vi "Logger.Stats.Fglb.vi"(4 "Time To":dbl, 6 "Time From":dbl, 7 "Action (get)":T2=enum."get", 8 "error in (no error)":errorcluster, 9 "dbg_NOK":dbl[](array[numeric]), 10 "dbg_OK":dbl[](array[numeric]), 11 "Variant":string) -> (0 "error out":errorcluster, 2 "Results":T1[](array[typedef]) {"Time From" format="%<%X %x>T"; "Time To" format="%<%X %x>T"})   [LabVIEW 2016]
uses:
  Logger.Stats.Fglb.Action.ctl
  Logger.Stats.Fglb.Result.ctl
  Global/ApplicationGlobal.vi
panel:
  out "dbg_var":string[](array[string])
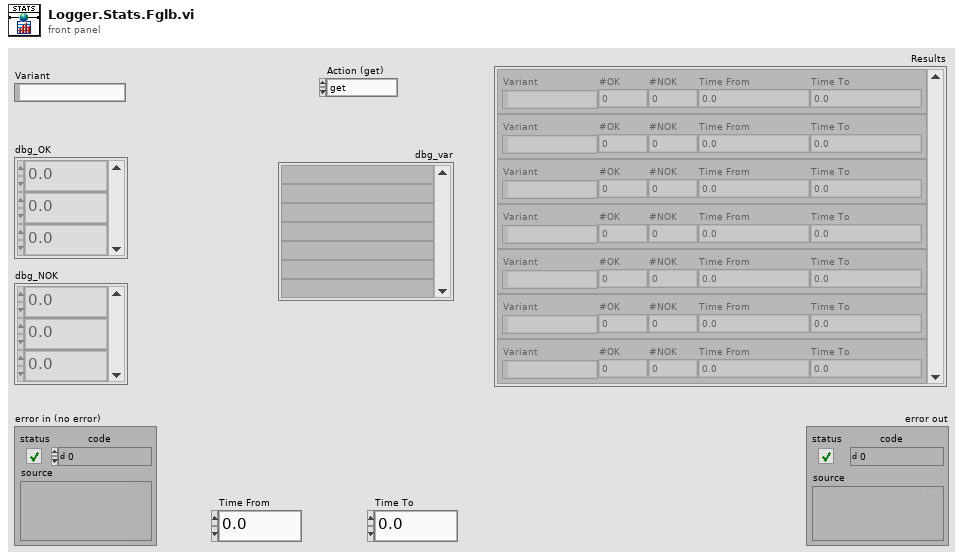
[diagram p1: front panel]
types:
  T1 = typedef "Logger.Stats.Fglb.Result.ctl" = cluster{"Variant":string, "#OK":i32, "#NOK":i32, "Time From":dbl, "Time To":dbl}
  T2 = typedef "Logger.Stats.Fglb.Action.ctl" = enum16{"init", "add", "get", "get all"}
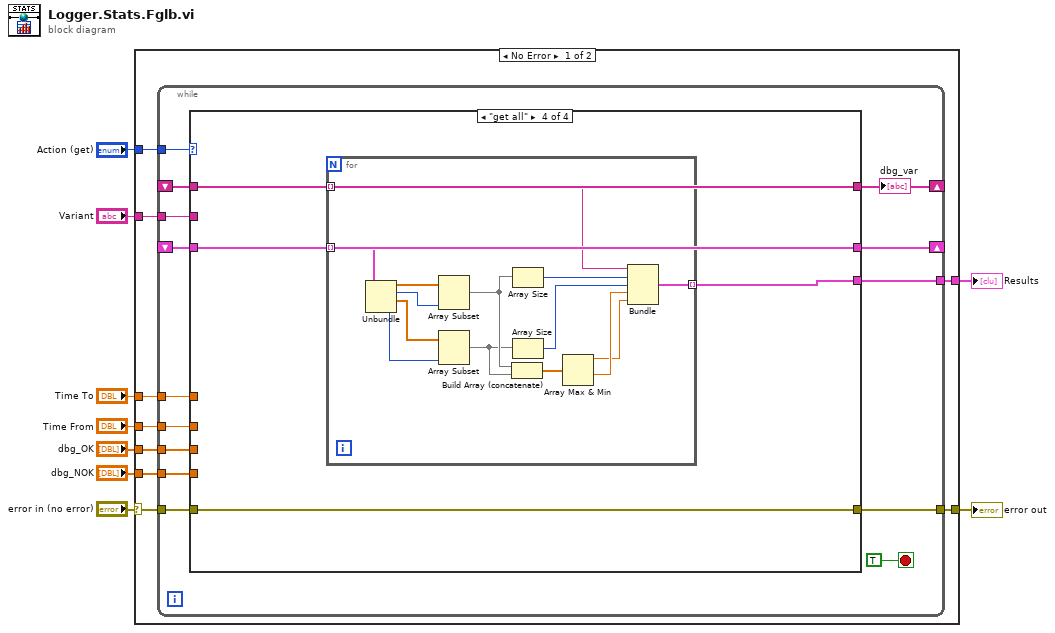
[diagram p0: block diagram]
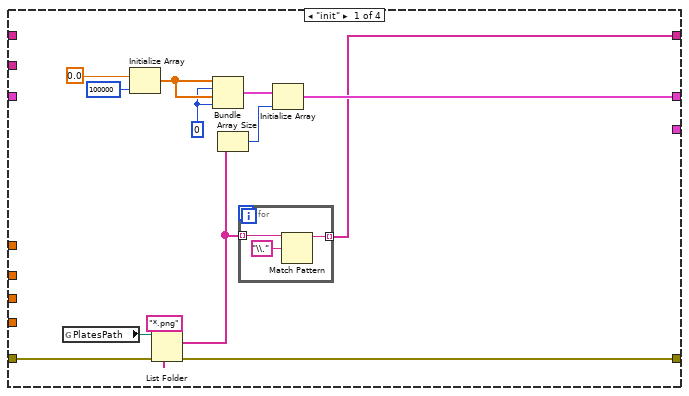
[diagram p2: hidden frame]
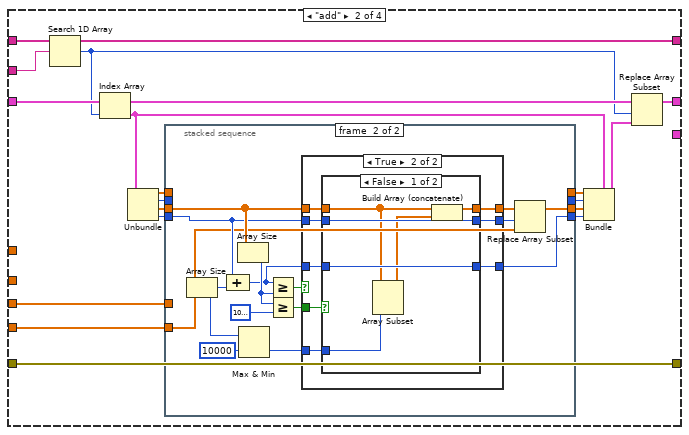
[diagram p3: hidden frame]
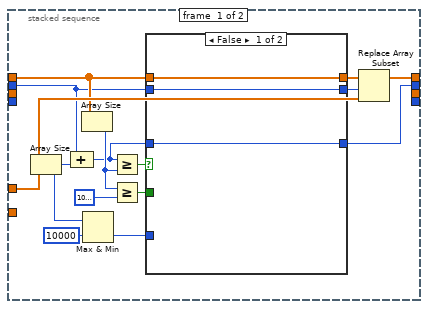
[diagram p4: hidden frame]
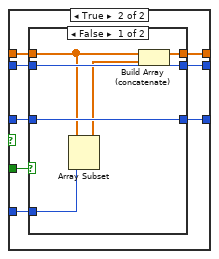
[diagram p5: hidden frame]
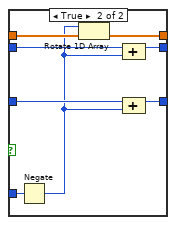
[diagram p6: hidden frame]
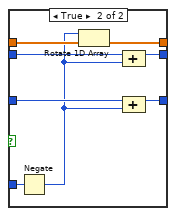
[diagram p8: hidden frame]
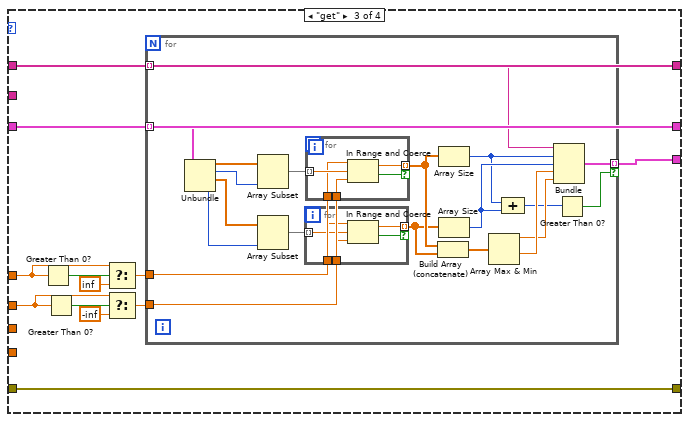
[diagram p9: hidden frame]
diagram:
  n1 = case shown="No Error" "error in (no error)" {
    selector: "error in (no error)" -> [w17 w207]
    tunnel: "Action (get)" -> [w18 _]
    tunnel: [w16 w207] -> w7
    tunnel: "Variant" -> [w15 _]
    tunnel: "dbg_OK" -> [w14 _]
    tunnel: "dbg_NOK" -> [w13 _]
    tunnel: "Time From" -> [w12 _]
    tunnel: "Time To" -> [w11 _]
    tunnel: [w10 _] -> w1
    frame No Error {
      n2 = while {
        tunnel: w18 -> [w32]
        shift-right: [w29] -> _
        shift-left: _ -> [w30]
        tunnel: w17 -> [w28]
        shift-right: [w27] -> _
        shift-left: _ -> [w26]
        tunnel: [w25] -> w16
        tunnel: w15 -> [w24]
        tunnel: w14 -> [w23]
        tunnel: w13 -> [w22]
        tunnel: w12 -> [w21]
        tunnel: w11 -> [w20]
        tunnel: [w19] -> w10
        stop <- TRUE stop-if-true
        n3 = case shown="\"get all\"" w32 {
          tunnel: w30 -> [_ w65 w147 w189]
          tunnel: [w33 w65 w147 w189] -> w29
          tunnel: w28 -> [w42 w51 w158 w192]
          tunnel: [w37 w63 w149 w191] -> w27
          tunnel: w26 -> [_ w64 w149 w191]
          tunnel: [w36 w51 w158 w192] -> w25
          tunnel: w24 -> [_ w66 _ _]
          tunnel: w23 -> [_ w58 _ _]
          tunnel: w22 -> [_ w52 _ _]
          tunnel: w21 -> [_ _ w157 _]
          tunnel: w20 -> [_ _ w152 _]
          tunnel: [_ _ w148 w190] -> w19
          frame "init" {
            w43 = 0
            n4 = global read "ApplicationGlobal.vi" "PlatesPath"() -> (w40:path)
            n5 = Initialize Array(0.0 ("Time Stamp"), 100000 ("dimension size")) -> (w44:dbl[])
            n6 = List Folder(path=w40, pattern="*.png" ("string"), error in=w42) -> (filenames=w34:string[], error out=w36:errorcluster)  [unwired: 1 in, 2 out]
            n7 = Bundle(w44, w43, w44, w43) -> (w39:cluster{dbl[], i32, dbl[], i32})  [unwired: 1 in]
            n8 = Array Size(array=w34) -> (size(s)=w38:i32)
            n9 = for {
              tunnel: w34 -> [w48] mode=indexing
              tunnel: [w46] -> w33 mode=indexing
              n10 = Match Pattern(string=w48, regular expression="\\.") -> (before substring=w46:string)  [unwired: 1 in, 3 out]
            }
            n11 = Initialize Array(w39, w38) -> (w37:cluster{dbl[], i32, dbl[], i32}[])
          }
          frame "add" {
            n12 = Search 1D Array(1D array=w65, element=w66) -> (index of element=w62:i32)  [unwired: 1 in]
            n13 = Index Array(array=w64, index=w62) -> (element=w61:cluster{dbl[], i32, dbl[], i32})
            n14 = Unbundle(w61) -> (w57:dbl[], w56:i32, w54:dbl[], w53:i32)
            n15 = stacked-sequence {
              tunnel: [w81 _] -> w59
              tunnel: w58 -> [w72 _]
              tunnel: w57 -> [w71 _]
              tunnel: w56 -> [w70 _]
              tunnel: [w73 _] -> w55
              tunnel: w54 -> [_ w109]
              tunnel: w53 -> [_ w108]
              tunnel: w52 -> [_ w107]
              tunnel: [_ w111] -> w50
              tunnel: [_ w110] -> w49
              frame #0 {
                n16 = Array Size(array=w72) -> (size(s)=w69:i32)
                n17 = Compound Arithmetic op=ADD(w70, w69) -> (w74:i32)
                n18 = Array Size(array=w71) -> (size(s)=w80:i32)
                n19 = Max & Min(x=w69, y=10000 ("dimension size")) -> (min(x,y)=w67:i32)  [unwired: 1 out]
                n20 = Greater Or Equal?(x=w74, y=w80) -> (x >= y?=w78:bool)
                n21 = Greater Or Equal?(x=w80, y=1000000) -> (x >= y?=w76:bool)
                n22 = case shown="False" w78 {
                  tunnel: w71 -> [w84 w92]
                  tunnel: [w84 w91] -> w77
                  tunnel: w76 -> [_ w90]
                  tunnel: w70 -> [w83 w89]
                  tunnel: [w83 w86] -> w75
                  tunnel: w74 -> [w82 w88]
                  tunnel: [w82 w87] -> w73
                  tunnel: w67 -> [_ w85]
                  frame False {
                  }
                  frame True {
                    n23 = case shown="False" w90 {
                      tunnel: w92 -> [w94 w106]
                      tunnel: [w98 w105] -> w91
                      tunnel: w89 -> [w96 w101]
                      tunnel: w88 -> [w97 w103]
                      tunnel: [w97 w102] -> w87
                      tunnel: [w96 w99] -> w86
                      tunnel: w85 -> [w95 w104]
                      frame False {
                        n24 = Array Subset(array=w94, length=w95) -> (w93:dbl[])  [unwired: 1 in]
                        n25 = Build Array (concatenate)(w94, w93) -> (w98:dbl[])
                      }
                      frame True {
                        n26 = Negate(x=w104) -> (-x=w100:i32)
                        n27 = Rotate 1D Array(1:w106, 2:w100) -> (0:w105:dbl[])
                        n28 = Compound Arithmetic op=ADD(w101, w100) -> (w99:i32)
                        n29 = Compound Arithmetic op=ADD(w103, w100) -> (w102:i32)
                      }
                    }
                  }
                }
                n30 = Replace Array Subset(array=w77, new element=w72, index=w75) -> (w81:dbl[])
              }
              frame #1 {
                n31 = Array Size(array=w107) -> (size(s)=w114:i32)
                n32 = Compound Arithmetic op=ADD(w108, w114) -> (w115:i32)
                n33 = Array Size(array=w109) -> (size(s)=w121:i32)
                n34 = Max & Min(x=w114, y=10000 ("dimension size")) -> (min(x,y)=w112:i32)  [unwired: 1 out]
                n35 = Greater Or Equal?(x=w115, y=w121) -> (x >= y?=w119:bool)
                n36 = Greater Or Equal?(x=w121, y=1000000) -> (x >= y?=w117:bool)
                n37 = case shown="True" w119 {
                  tunnel: w109 -> [w124 w132]
                  tunnel: [w124 w131] -> w118
                  tunnel: w117 -> [_ w130]
                  tunnel: w108 -> [w123 w129]
                  tunnel: [w123 w126] -> w116
                  tunnel: w115 -> [w122 w128]
                  tunnel: [w122 w127] -> w111
                  tunnel: w112 -> [_ w125]
                  frame False {
                  }
                  frame True {
                    n38 = case shown="False" w130 {
                      tunnel: w132 -> [w134 w146]
                      tunnel: [w138 w145] -> w131
                      tunnel: w129 -> [w136 w141]
                      tunnel: w128 -> [w137 w143]
                      tunnel: [w137 w142] -> w127
                      tunnel: [w136 w139] -> w126
                      tunnel: w125 -> [w133 w144]
                      frame False {
                        n39 = Array Subset(array=w134, length=w133) -> (w135:dbl[])  [unwired: 1 in]
                        n40 = Build Array (concatenate)(w134, w135) -> (w138:dbl[])
                      }
                      frame True {
                        n41 = Negate(x=w144) -> (-x=w140:i32)
                        n42 = Rotate 1D Array(1:w146, 2:w140) -> (0:w145:dbl[])
                        n43 = Compound Arithmetic op=ADD(w141, w140) -> (w139:i32)
                        n44 = Compound Arithmetic op=ADD(w143, w140) -> (w142:i32)
                      }
                    }
                  }
                }
                n45 = Replace Array Subset(array=w118, new element=w107, index=w116) -> (w110:dbl[])
              }
            }
            n46 = Bundle(cluster=w61, w59, w55, w49, w50) -> (w60:cluster{dbl[], i32, dbl[], i32})
            n47 = Replace Array Subset(array=w64, new element=w60, index=w62) -> (w63:cluster{dbl[], i32, dbl[], i32}[])
          }
          frame "get" {
            n48 = Greater Than 0?(x=w152) -> (x > 0?=w153:bool)
            n49 = Greater Than 0?(x=w157) -> (x > 0?=w156:bool)
            n50 = Select(t=w152, s=w153, f=inf) -> (s? t:f=w151:dbl)
            n51 = Select(t=w157, s=w156, f=-inf) -> (s? t:f=w150:dbl)
            n52 = for {
              tunnel: w151 -> [w172]
              tunnel: w150 -> [w171]
              tunnel: [w170] -> w148 mode=indexing if=w159
              tunnel: w149 -> [w169] mode=indexing
              tunnel: w147 -> [w165] mode=indexing
              n53 = Unbundle(w169) -> (w178:dbl[], w177:i32, w176:dbl[], w175:i32)
              n54 = Array Subset(array=w178, length=w177) -> (w174:dbl[])  [unwired: 1 in]
              n55 = Array Subset(array=w176, length=w175) -> (w173:dbl[])  [unwired: 1 in]
              n56 = for {
                tunnel: w173 -> [w183] mode=indexing
                tunnel: w172 -> [w182]
                tunnel: w171 -> [w181]
                tunnel: [w180] -> w163 mode=indexing if=w179
                n57 = In Range and Coerce(upper limit=w182, x=w183, lower limit=w181) -> (coerced(x)=w180:dbl, In Range?=w179:bool)
              }
              n58 = for {
                tunnel: w174 -> [w188] mode=indexing
                tunnel: w172 -> [w187]
                tunnel: w171 -> [w186]
                tunnel: [w185] -> w164 mode=indexing if=w184
                n59 = In Range and Coerce(upper limit=w187, x=w188, lower limit=w186) -> (coerced(x)=w185:dbl, In Range?=w184:bool)
              }
              n60 = Build Array (concatenate)(w164, w163) -> (w168:dbl[])
              n61 = Array Size(array=w164) -> (size(s)=w161:i32)
              n62 = Array Size(array=w163) -> (size(s)=w162:i32)
              n63 = Array Max & Min(array=w168) -> (max value=w166:dbl, min value=w167:dbl)  [unwired: 2 out]
              n64 = Compound Arithmetic op=ADD(w161, w162) -> (w160:i32)
              n65 = Bundle(w165, w161, w162, w167, w166) -> (w170:cluster{string, i32, i32, dbl, dbl})  [unwired: 1 in]
              n66 = Greater Than 0?(x=w160) -> (x > 0?=w159:bool)
            }
          }
          frame "get all" {
            n67 = for {
              tunnel: [w200] -> w190 mode=indexing
              tunnel: w191 -> [w199] mode=indexing
              tunnel: w189 -> [w195] mode=indexing
              n68 = Unbundle(w199) -> (w206:dbl[], w205:i32, w204:dbl[], w203:i32)
              n69 = Array Subset(array=w206, length=w205) -> (w194:dbl[])  [unwired: 1 in]
              n70 = Array Subset(array=w204, length=w203) -> (w193:dbl[])  [unwired: 1 in]
              n71 = Build Array (concatenate)(w194, w193) -> (w198:dbl[])
              n72 = Array Size(array=w194) -> (size(s)=w202:i32)
              n73 = Array Size(array=w193) -> (size(s)=w201:i32)
              n74 = Array Max & Min(array=w198) -> (max value=w196:dbl, min value=w197:dbl)  [unwired: 2 out]
              n75 = Bundle(w195, w202, w201, w197, w196) -> (w200:cluster{string, i32, i32, dbl, dbl})  [unwired: 1 in]
            }
          }
        }
        "dbg_var" <- w29
      }
    }
    frame Error {
    }
  }
  "error out" <- w7
  "Results" <- w1
